vi "Simulator Stop.vi"() -> ()   [LabVIEW 2017]
uses:
  E:/UPWORK/Laser Tool/Laser/project/data/Thorlabs.MotionControl.DeviceManagerCLI.dll
  project/data/Thorlabs.MotionControl.DeviceManagerCLI.dll
panel:
  out "error out":errorcluster
  in  "serialNo":string="97000001"
  # "STOP"
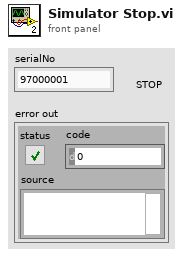
[diagram p1: front panel]
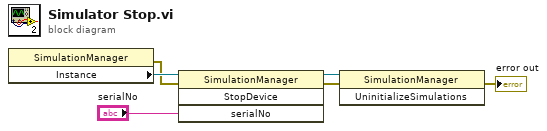
[diagram p0: block diagram]
diagram:
  n1 = property class="SimulationManager"() -> (error out=w5:errorcluster, "Instance"=w6:refnum<k24>)  [unwired: 2 in, 1 out]
  n2 = invoke class="SimulationManager" method="StopDevice"(reference=w6, error in=w5, "serialNo"="serialNo") -> (reference out=w2:refnum<k24>, error out=w3:errorcluster)  [unwired: 1 in, 2 out]
  n3 = invoke class="SimulationManager" method="UninitializeSimulations"(reference=w2, error in=w3) -> (error out=→"error out":errorcluster)  [unwired: 1 in, 2 out]
